vi "main.vi"() -> ()   [LabVIEW 2020]
doc: "This VI is used as the driver for the queue to work. It performs the operations in the queue."
uses:
  Typedef's/Data_Cluster.ctl
  Typedef's/Q_Operations.ctl
  <vilib>/Utility/error.llb/DialogType.ctl
  Typedef's/Bewarage_Out_Level.ctl
  Typedef's/Content_Level.ctl
  <vilib>/Utility/config.llb/NI_LVConfig.lvlib
  Typedef's/Timer_Details.ctl
  Typedef's/Operation_Indication.ctl
  Typedef's/Low_Level_Indications.ctl
  <vilib>/Utility/config.llb/Write Key (I32).vi
  <vilib>/Utility/config.llb/Config Data RefNum.ctl
  <vilib>/Utility/config.llb/Read Key (I32).vi
  <vilib>/Utility/config.llb/Read Key (Boolean).vi
  <vilib>/Utility/config.llb/Read Key (U32).vi
  <vilib>/Utility/config.llb/Write Key (U32).vi
panel:
  out "Error Out":errorcluster
  in  "Error In":errorcluster
  in  "Power":bool
  out "Total Cups":u32
  out "Elapsed Time":i32
  out "Dispensing":bool
  out "Brewing":bool
  out "Grinding":bool
  out "Heating":bool
  out "Purging":bool
  out "Dispenser":i32(slide) min=0 max=60 step=1 scale=0.0..60.0
  out "Chamber":i32(slide) min=0 max=60 step=1 scale=0.0..60.0
  out "Low Milk":bool
  out "Low Bean":bool
  out "Low Water":bool
  out "Milk Level":i32(slide) min=0 max=100 step=1 scale=0.0..100.0
  out "Bean Level":i32(slide) min=0 max=100 step=1 scale=0.0..100.0
  out "Water Level":i32(slide) min=0 max=100 step=1 scale=0.0..100.0
  in  "Bewarage":i32(knob) min=0 max=2 step=1 scale=0.0..2.0
  in  "Carafe":bool
  in  "1 Cup":bool
  # "Description: \n-> Only after power on. Make the button press\nto make coffee"
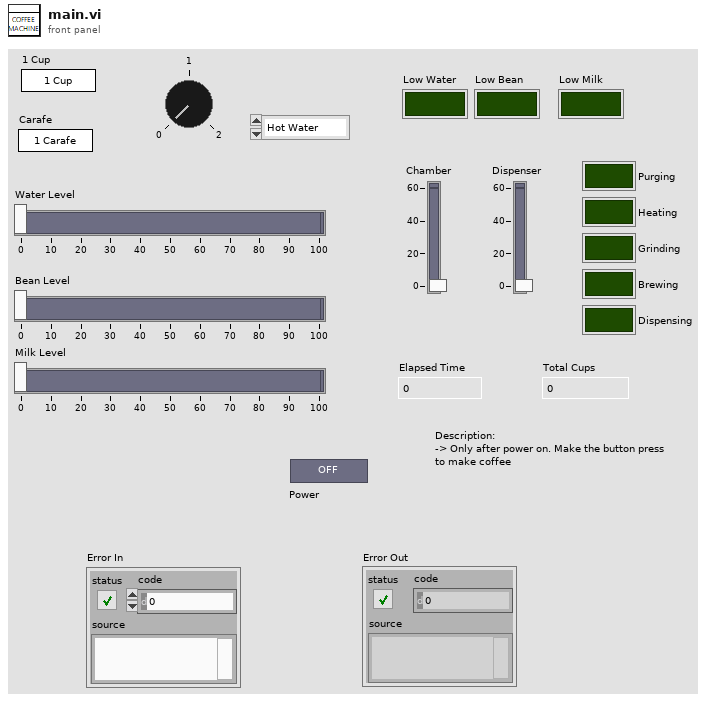
[diagram p1: front panel]
types:
  T1 = typedef "Q_Operations.ctl" = enum16{"Create Q", "Enqueue ", "Dequeue", "Enqueue N ele", "Enstack N ele", "Flush Q", "Destroy Q"}
  T2 = typedef "Data_Cluster.ctl" = cluster{"Cup":bool, "Bewarage":dbl, "Carafe":bool, "Power":bool, "Content Levels":T3, "Beware Out Level":T4, "Timer Operations":T5, "Cups Count":u32, "Bewarage Low Level":i32, "Sequence Array":string[], "Operation Indication":T6, "Bewarage Selection":string, "Low Level Indications":T7, "Config Data Ref":T8}
  T3 = typedef "Content_Level.ctl" = cluster{"Water Level":i32, "Bean Level":i32, "Milk Level":i32}
  T4 = typedef "Bewarage_Out_Level.ctl" = cluster{"Dispenser":i32, "Chamber":i32}
  T5 = typedef "Timer_Details.ctl" = cluster{"Set Time":dbl, "Prev Time":dbl, "Elapsed Time":dbl, "Start?":bool, "Paused?":bool}
  T6 = typedef "Operation_Indication.ctl" = cluster{"Heating":bool, "Grinding":bool, "Dispensing":bool, "Purging":bool, "Brewing":bool}
  T7 = typedef "Low_Level_Indications.ctl" = cluster{"Low Water":bool, "Low Milk":bool, "Low Bean":bool}
  T8 = typedef "NI_LVConfig.lvlib/Config Data RefNum.ctl" = refnum<k1>
  T9 = typedef "DialogType.ctl" = u16
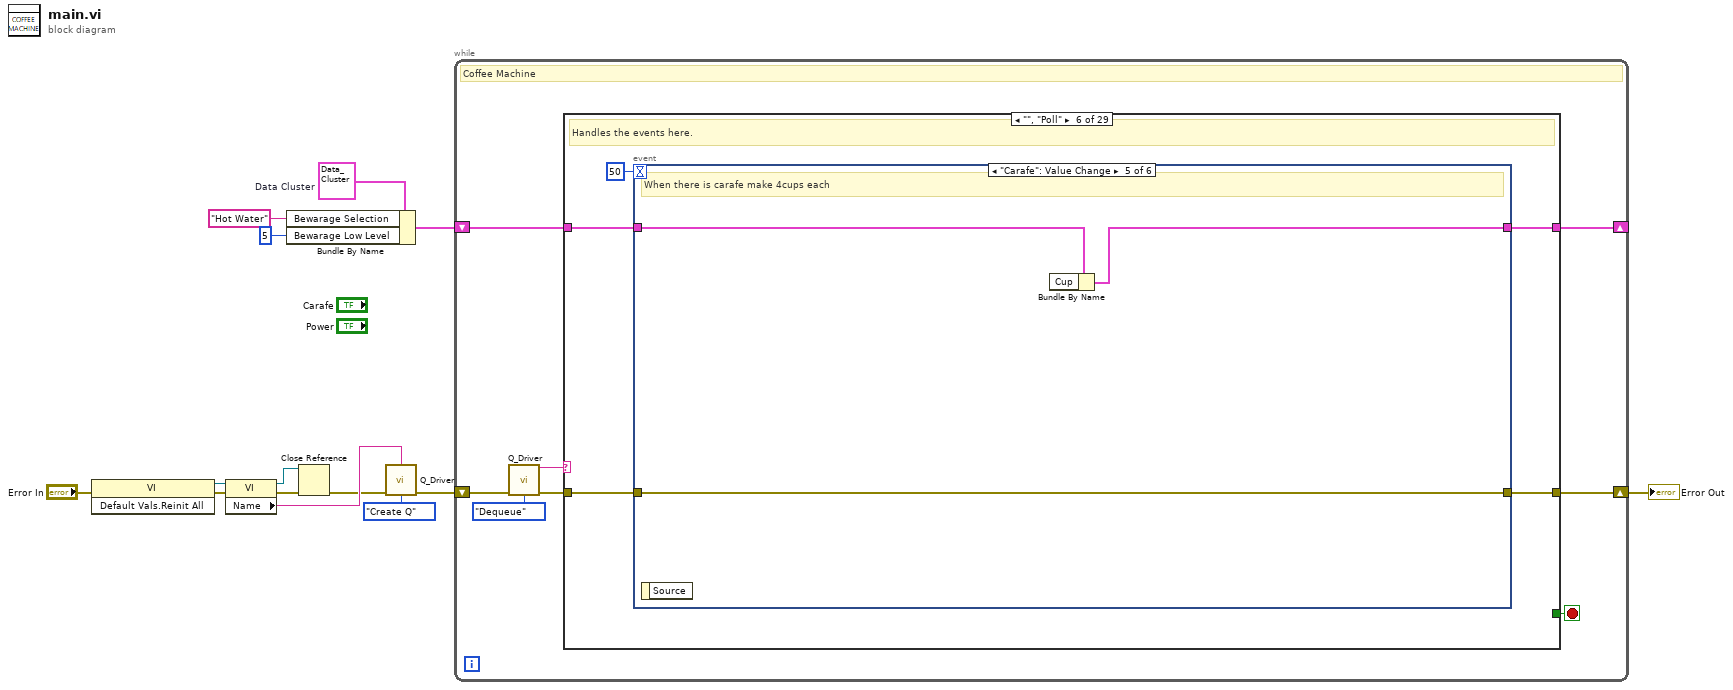
[diagram p0: block diagram]
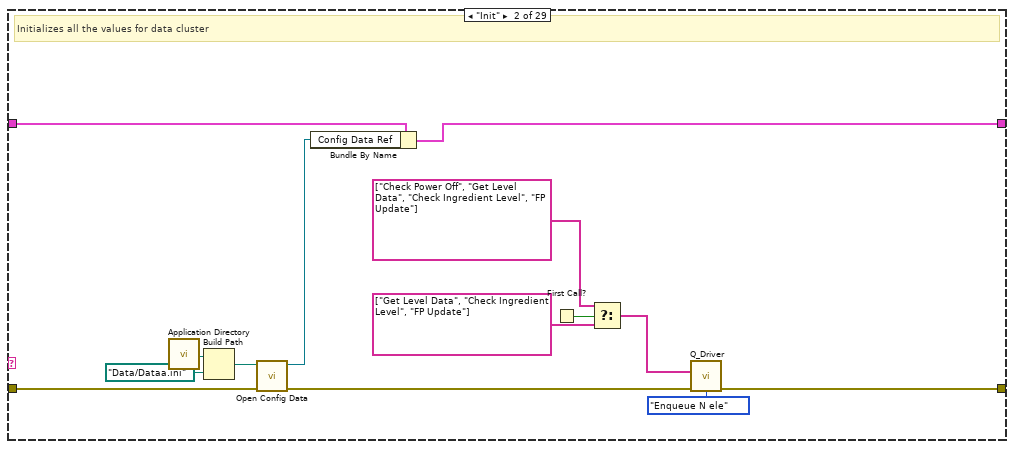
[diagram p3: hidden frame]
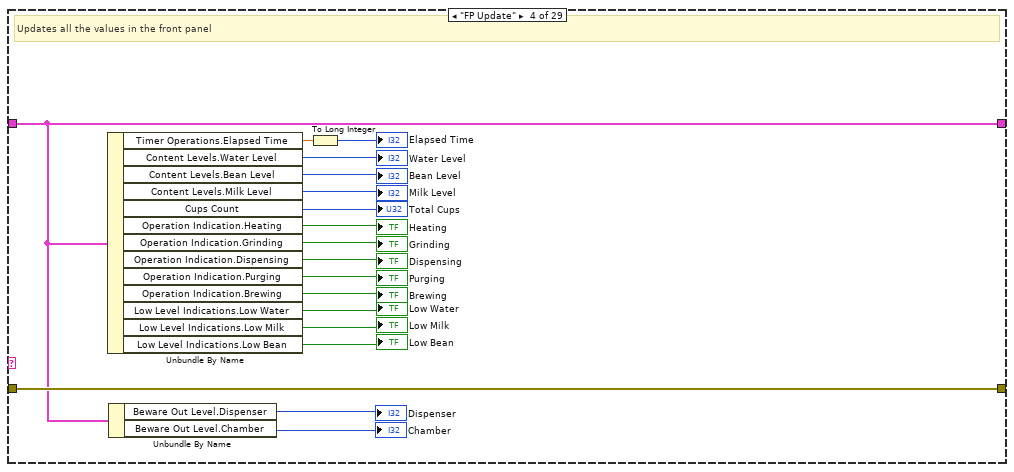
[diagram p5: hidden frame]
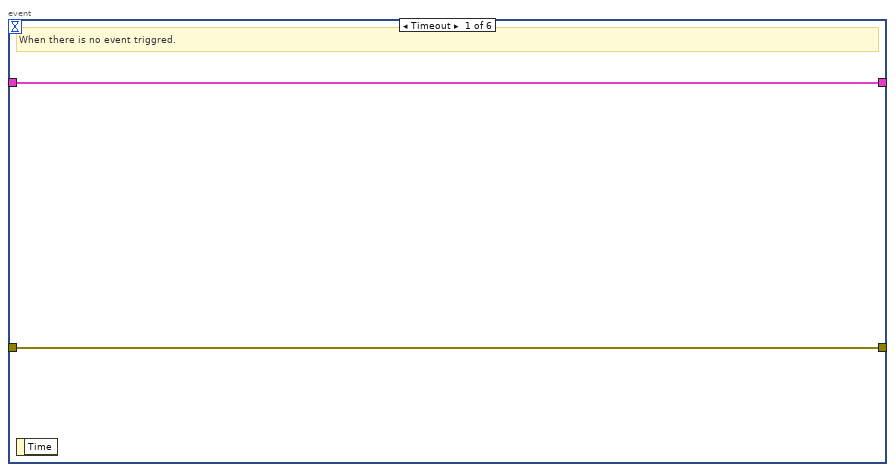
[diagram p7: hidden frame]
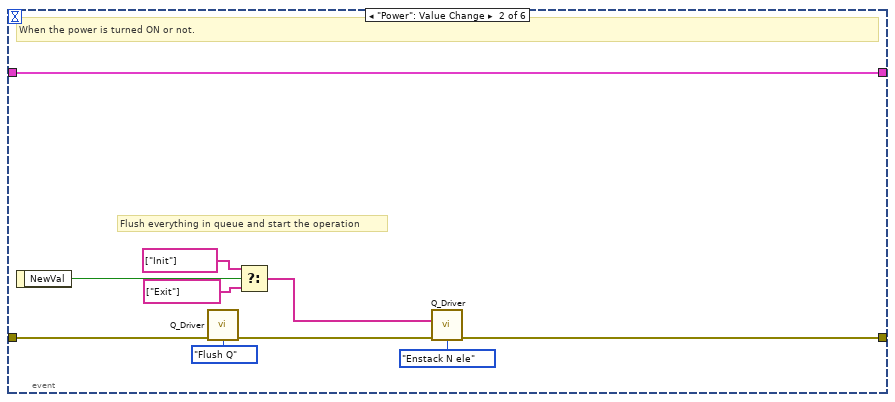
[diagram p8: hidden frame]
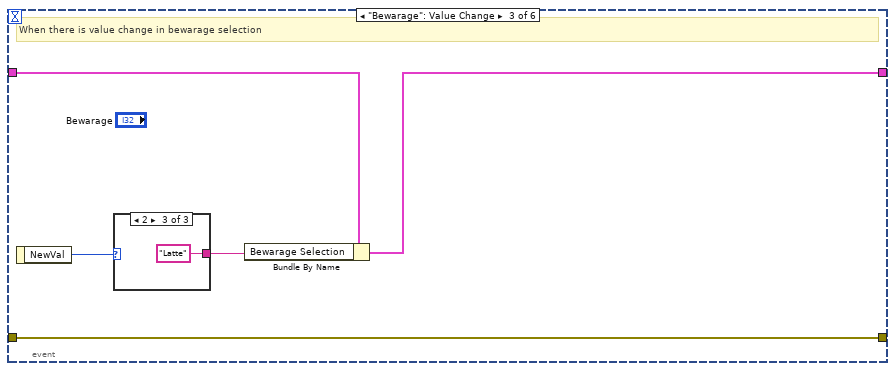
[diagram p9: hidden frame]
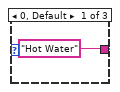
[diagram p10: hidden frame]
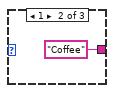
[diagram p11: hidden frame]
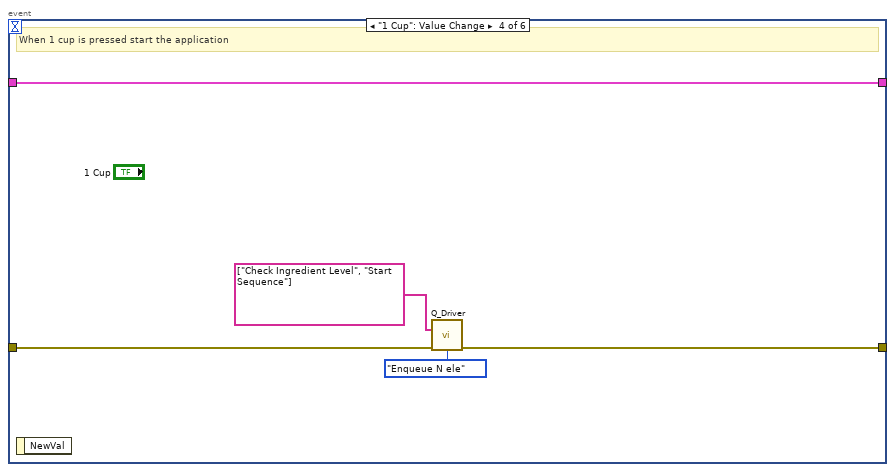
[diagram p12: hidden frame]
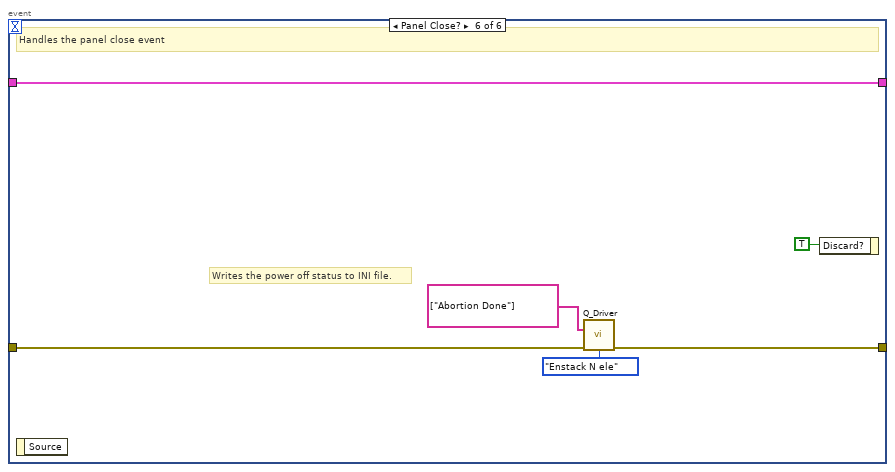
[diagram p13: hidden frame]
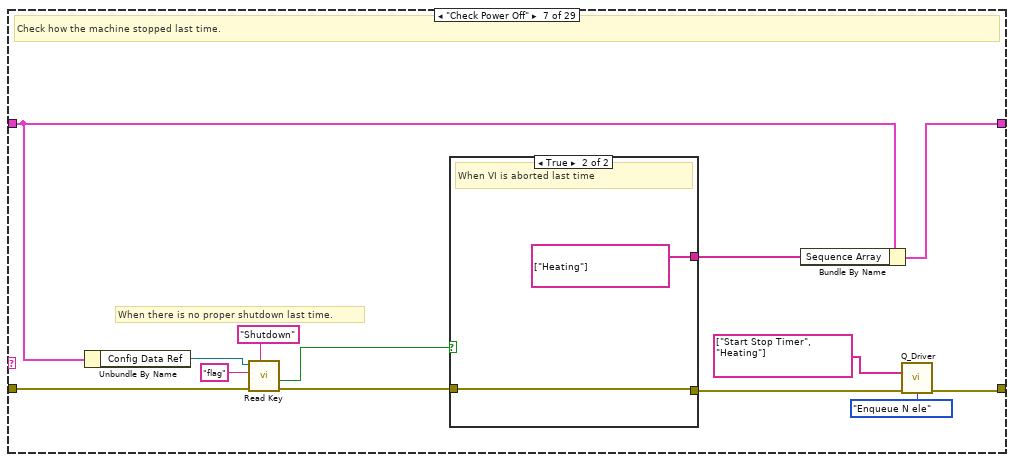
[diagram p14: hidden frame]
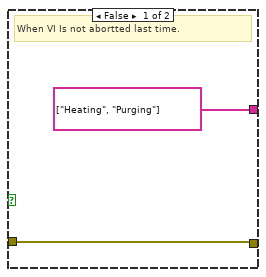
[diagram p15: hidden frame]
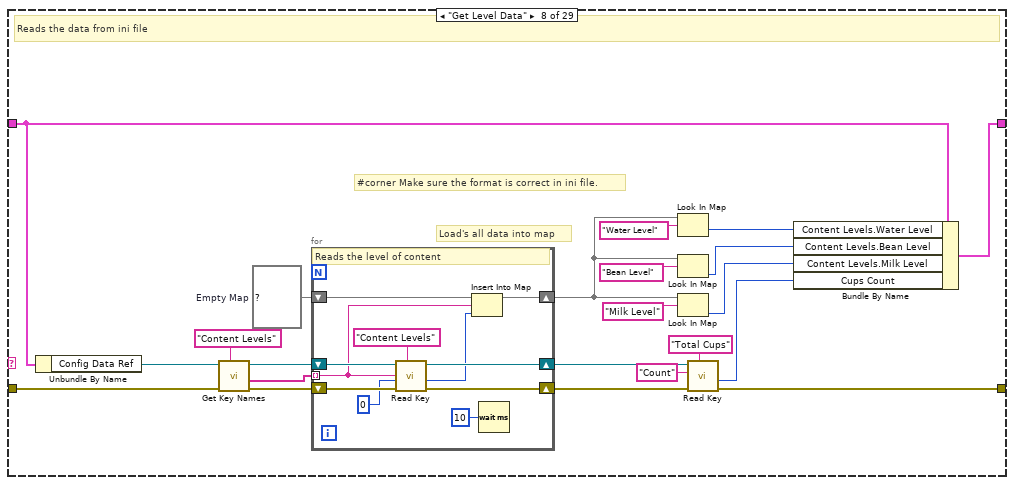
[diagram p16: hidden frame]
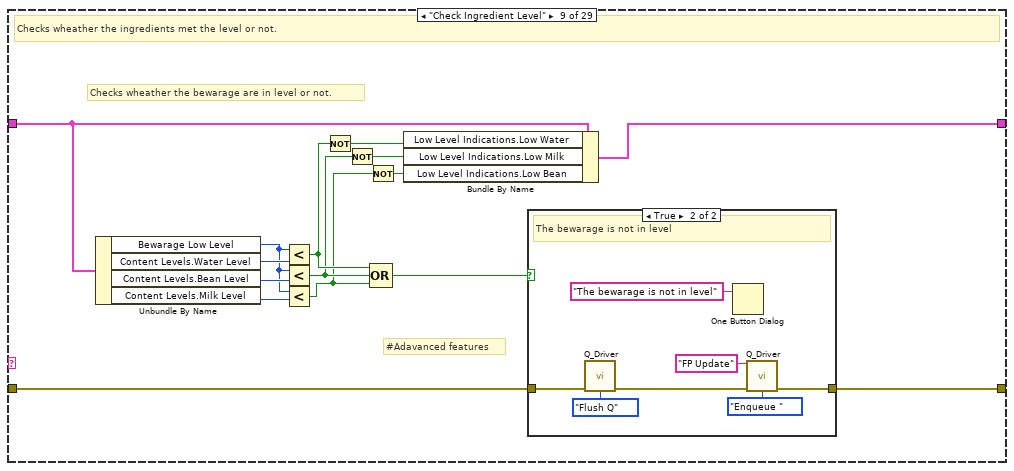
[diagram p17: hidden frame]
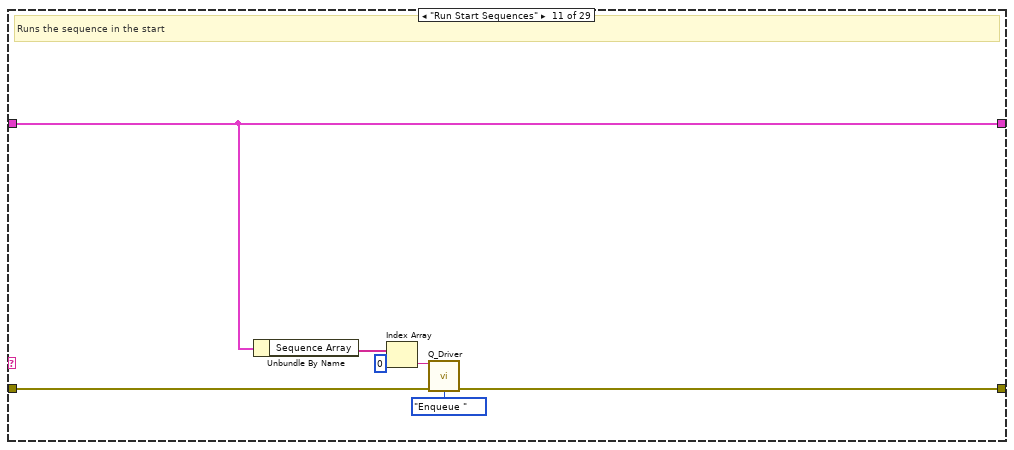
[diagram p20: hidden frame]
diagram:
  w9 = T2 {"Cup"=FALSE, "Bewarage"=0.0, "Carafe"=FALSE, "Power"=FALSE, "Content Levels"={"Water Level"=0, "Bean Level"=0, "Milk Level"=0}, "Beware Out Level"={"Dispenser"=0, "Chamber"=0}, "Timer Operations"={"Set Time"=0.0, "Prev Time"=0.0, "Elapsed Time"=0.0, "Start?"=FALSE, "Paused?"=FALSE}, "Cups Count"=0, "Bewarage Low Level"=30, "Sequence Array"=[], "Operation Indication"={"Heating"=FALSE, "Grinding"=FALSE, "Dispensing"=FALSE, "Purging"=FALSE, "Brewing"=FALSE}, "Bewarage Selection"="Hot Water", "Low Level Indications"={"Low Water"=FALSE, "Low Milk"=FALSE, "Low Bean"=FALSE}, "Config Data Ref"=refnum}  # Data Cluster
  n1 = invoke class="VI" method="Default Vals.Reinit All"(error in="Error In") -> (reference out=w4:refnum<vi>, error out=w5:errorcluster)  [unwired: 2 in, 1 out]
  n2 = property class="VI"(reference=w4, error in=w5) -> (reference out=w2:refnum<vi>, error out=w11:errorcluster, "Name"=w10:string)
  n3 = Bundle By Name(cluster=w9, "Bewarage Selection"="Hot Water", "Bewarage Low Level"=5) -> (w8:T2)
  n4 = Close Reference(reference=w2, error in (no error)=w11) -> (error out=w3:errorcluster)
  n5 = call "Q_Driver.vi"("Q Name"=w10, "Error In"=w3, "Operations"=Q_Operations."Create Q") -> ("Error Out"=w13:errorcluster)  [unwired: 11 in, 1 out]
  n6 = while {
    shift-right: [w21] -> w6
    shift-left: w13 -> [w22]
    shift-right: [w16] -> _
    shift-left: w8 -> [w17]
    stop <- w15 stop-if-true
    # "Coffee Machine"
    n7 = call "Q_Driver.vi"("Error In"=w22, "Operations"=Q_Operations."Dequeue") -> ("Dequeued Ele"=w18:string, "Error Out"=w20:errorcluster)  [unwired: 12 in]
    n8 = case shown="\"\", \"Poll\"" w18 {
      tunnel: w20 -> [w24 w37 w40 w58 w60 w65 w112 w138 w154 w174 w181 w193 w197 w207 w215 w242 w259 w278 w295 w338 w340 w349 w360 w379 w385 w387 w396 w405 w407]
      tunnel: [w24 w36 w40 w58 w60 w64 w102 w122 w153 w174 w177 w191 w198 w207 w210 w237 w258 w277 w290 w310 w340 w349 w351 w379 w382 w387 w390 w400 w407] -> w21
      tunnel: w17 -> [w23 w38 w39 w43 w59 w62 w104 w123 w164 w173 w180 w192 w205 w206 w216 w233 w256 w275 w293 w333 w339 w347 w359 w378 w380 w386 w395 w402 w406]
      tunnel: [w23 w34 w39 w43 w59 w61 w105 w127 w158 w173 w180 w189 w204 w206 w214 w241 w262 w281 w294 w326 w339 w348 w355 w378 w380 w386 w395 w402 w406] -> w16
      tunnel: [_ _ _ _ _ _ _ _ _ _ _ _ _ _ _ _ _ _ _ _ _ _ _ _ _ _ TRUE TRUE _] -> w15
      frame "/**** Initialization ****/" {
      }
      frame "Init" {
        # "Initializes all the values for data cluster"
        n9 = call <vilib>:"Application Directory.vi"() -> ("Application Directory"=w31:path)
        n10 = Build Path(base path=w31, name or relative path=path "Data/Dataa.ini") -> (appended path=w30:path)
        n11 = call <vilib>:"Open Config Data.vi"("error in (no error)"=w37, "configuration file path"=w30) -> ("error out"=w33:errorcluster, "refnum"=w29:T8)  [unwired: 7 in, 1 out]
        n12 = Bundle By Name(cluster=w38, "Config Data Ref"=w29) -> (w34:T2)
        n13 = First Call?() -> (First Call?: T/F=w28:bool)
        n14 = Select(t=string[] ["Check Power Off", "Get Level Data", "Check Ingredient Level", "FP Update"], s=w28, f=string[] ["Get Level Data", "Check Ingredient Level", "FP Update"]) -> (s? t:f=w25:string[])
        n15 = call "Q_Driver.vi"("States[]"=w25, "Error In"=w33, "Operations"=Q_Operations."Enqueue N ele") -> ("Error Out"=w36:errorcluster)  [unwired: 11 in, 1 out]
      }
      frame "/***** FP Related ****/" {
      }
      frame "FP Update" {
        # "Updates all the values in the front panel"
        n16 = Unbundle By Name(w43) -> ("Timer Operations.Elapsed Time"=w48:dbl, "Content Levels.Water Level"=→"Water Level":i32, "Content Levels.Bean Level"=→"Bean Level":i32, "Content Levels.Milk Level"=→"Milk Level":i32, "Cups Count"=→"Total Cups":u32, "Operation Indication.Heating"=→"Heating":bool, "Operation Indication.Grinding"=→"Grinding":bool, "Operation Indication.Dispensing"=→"Dispensing":bool, "Operation Indication.Purging"=→"Purging":bool, "Operation Indication.Brewing"=→"Brewing":bool, "Low Level Indications.Low Water"=→"Low Water":bool, "Low Level Indications.Low Milk"=→"Low Milk":bool, "Low Level Indications.Low Bean"=→"Low Bean":bool)
        n17 = Unbundle By Name(w43) -> ("Beware Out Level.Dispenser"=→"Dispenser":i32, "Beware Out Level.Chamber"=→"Chamber":i32)
        n18 = To Long Integer(number=w48) -> (32bit integer=→"Elapsed Time":i32)
      }
      frame "/***** Events and Functionalities *****/" {
      }
      frame "", "Poll" {
        # "Handles the events here."
        n19 = event shown="[4] \"Carafe\": Value Change" {
          selector: _ -> [_ _ _ _ _ _]
          dyn-events: _ -> [_ _ _ _ _ _]
          timeout: 50 -> [_ _ _ _ _ _]
          tunnel: [w67 w72 w82 w88 w93 w97] -> w64
          tunnel: w65 -> [w67 w77 w82 w90 w93 w99]
          tunnel: [w66 w76 w79 w89 w91 w94] -> w61
          tunnel: w62 -> [w66 w76 w81 w89 w92 w94]
          event Timeout {
            # "When there is no event triggred."
            n20 = event-data() -> ()  [unwired: 1 in, 1 out]
          }
          event "Power": Value Change {
            # "Flush everything in queue and start the operation"
            # "When the power is turned ON or not."
            n21 = event-data() -> ("NewVal"=w75:bool)  [unwired: 1 in]
            n22 = call "Q_Driver.vi"("Error In"=w77, "Operations"=Q_Operations."Flush Q") -> ("Error Out"=w69:errorcluster)  [unwired: 12 in, 1 out]
            n23 = Select(t=string[] ["Init"], s=w75, f=string[] ["Exit"]) -> (s? t:f=w70:string[])
            n24 = call "Q_Driver.vi"("States[]"=w70, "Error In"=w69, "Operations"=Q_Operations."Enstack N ele") -> ("Error Out"=w72:errorcluster)  [unwired: 11 in, 1 out]
          }
          event "Bewarage": Value Change {
            # "When there is value change in bewarage selection"
            n25 = event-data() -> ("NewVal"=w80:i32)  [unwired: 1 in]
            n26 = case shown="2" w80 {
              tunnel: ["Hot Water" "Coffee" "Latte"] -> w78
              frame 0, Default {
              }
              frame 1 {
              }
              frame 2 {
              }
            }
            n27 = Bundle By Name(cluster=w81, "Bewarage Selection"=w78) -> (w79:T2)
          }
          event "1 Cup": Value Change {
            # "When 1 cup is pressed start the application"
            n28 = event-data() -> ()  [unwired: 1 in, 1 out]
            n29 = call "Q_Driver.vi"("States[]"=string[] ["Check Ingredient Level", "Start Sequence"], "Error In"=w90, "Operations"=Q_Operations."Enqueue N ele") -> ("Error Out"=w88:errorcluster)  [unwired: 11 in, 1 out]
          }
          event "Carafe": Value Change {
            # "When there is carafe make 4cups each"
            n30 = event-data() -> ()  [unwired: 1 in, 1 out]
            n31 = Bundle By Name(cluster=w92) -> (w91:T2)  [unwired: 1 in]
          }
          event Panel Close? {
            # "Writes the power off status to INI file."
            # "Handles the panel close event"
            n32 = event-data() -> ()  [unwired: 1 in, 1 out]
            n33 = call "Q_Driver.vi"("States[]"=string[] ["Abortion Done"], "Error In"=w99, "Operations"=Q_Operations."Enstack N ele") -> ("Error Out"=w97:errorcluster)  [unwired: 11 in, 1 out]
            n34 = event-data("Discard?"=TRUE) -> ()  [unwired: 1 in, 1 out]
          }
        }
      }
      frame "Check Power Off" {
        # "When there is no proper shutdown last time."
        # "Check how the machine stopped last time."
        n35 = Unbundle By Name(w104) -> ("Config Data Ref"=w108:T8)
        n36 = call-poly <vilib>:"Read Key.vi"("section"="Shutdown", "error in (no error)"=w112, "key"="flag", "refnum"=w108) -> ("error out"=w107:errorcluster, "value"=w109:bool)  [unwired: 4 in, 2 out]
        n37 = case shown="True" w109 {
          tunnel: [w114 w116] -> w106
          tunnel: w107 -> [w114 w116]
          tunnel: [string[] ["Heating", "Purging"] ("Sequence Array") string[] ["Heating"] ("Sequence Array")] -> w103
          frame False {
            # "When VI Is not abortted last time."
          }
          frame True {
            # "When VI is aborted last time"
          }
        }
        n38 = Bundle By Name(cluster=w104, "Sequence Array"=w103) -> (w105:T2)
        n39 = call "Q_Driver.vi"("States[]"=string[] ["Start Stop Timer", "Heating"], "Error In"=w106, "Operations"=Q_Operations."Enqueue N ele") -> ("Error Out"=w102:errorcluster)  [unwired: 11 in, 1 out]
      }
      frame "Get Level Data" {
        w133 = map{string, i32} {}  # Empty Map
        # "Load's all data into map"
        # "#corner Make sure the format is correct in ini file."
        # "Reads the data from ini file"
        n40 = Unbundle By Name(w123) -> ("Config Data Ref"=w117:T8)
        n41 = call <vilib>:"Get Key Names.vi"("section"="Content Levels", "error in (no error)"=w138, "refnum"=w117) -> ("error out"=w137:errorcluster, "key names"=w135:string[], "refnum out"=w134:T8)  [unwired: 5 in, 1 out]
        n42 = for {
          shift-right: [w148] -> w136
          shift-left: w137 -> [w149]
          tunnel: w135 -> [w142] mode=indexing
          shift-right: [w145] -> w121
          shift-left: w134 -> [w146]
          shift-right: [w140] -> w128
          shift-left: w133 -> [w143]
          # "Reads the level of content"
          n43 = call-poly <vilib>:"Read Key.vi"("section"="Content Levels", "error in (no error)"=w149, "default value"=0, "key"=w142, "refnum"=w146) -> ("error out"=w148:errorcluster, "value"=w141:i32, "refnum out"=w145:T8)  [unwired: 3 in, 1 out]
          n44 = Insert Into Map(map in=w143, key=w142, value=w141) -> (map out=w140:map{string, i32})  [unwired: 2 out]
          n45 = Wait (ms)(milliseconds to wait=u32 10) -> ()  [unwired: 1 out]
        }
        n46 = Look In Map(map=w128, key="Water Level") -> (value=w126:i32)  [unwired: 1 in, 1 out]
        n47 = Look In Map(map=w128, key="Bean Level") -> (value=w125:i32)  [unwired: 1 in, 1 out]
        n48 = Look In Map(map=w128, key="Milk Level") -> (value=w124:i32)  [unwired: 1 in, 1 out]
        n49 = call-poly <vilib>:"Read Key.vi"("section"="Total Cups", "error in (no error)"=w136, "key"="Count", "refnum"=w121) -> ("error out"=w122:errorcluster, "value"=w120:u32)  [unwired: 4 in, 2 out]
        n50 = Bundle By Name(cluster=w123, "Content Levels.Water Level"=w126, "Content Levels.Bean Level"=w125, "Content Levels.Milk Level"=w124, "Cups Count"=w120) -> (w127:T2)
      }
      frame "Check Ingredient Level" {
        # "#Adavanced features"
        # "Checks wheather the bewarage are in level or not."
        # "Checks wheather the ingredients met the level or not."
        n51 = Unbundle By Name(w164) -> ("Bewarage Low Level"=w160:i32, "Content Levels.Water Level"=w163:i32, "Content Levels.Bean Level"=w162:i32, "Content Levels.Milk Level"=w161:i32)
        n52 = Less?(x=w160, y=w163) -> (x < y?=w157:bool)
        n53 = Less?(x=w160, y=w162) -> (x < y?=w156:bool)
        n54 = Less?(x=w160, y=w161) -> (x < y?=w155:bool)
        n55 = Not(x=w157) -> (.not. x?=w152:bool)
        n56 = Not(x=w156) -> (.not. x?=w151:bool)
        n57 = Not(x=w155) -> (.not. x?=w150:bool)
        n58 = Compound Arithmetic op=OR(w157, w156, w155) -> (w159:bool)
        n59 = Bundle By Name(cluster=w164, "Low Level Indications.Low Water"=w152, "Low Level Indications.Low Milk"=w151, "Low Level Indications.Low Bean"=w150) -> (w158:T2)
        n60 = case shown="True" w159 {
          tunnel: w154 -> [w165 w171]
          tunnel: [w165 w168] -> w153
          frame False {
            # "When they are in level"
          }
          frame True {
            # "The bewarage is not in level"
            n61 = call "Q_Driver.vi"("Error In"=w171, "Operations"=Q_Operations."Flush Q") -> ("Error Out"=w170:errorcluster)  [unwired: 12 in, 1 out]
            n62 = One Button Dialog(message="The bewarage is not in level") -> ()  [unwired: 1 in, 1 out]
            n63 = call "Q_Driver.vi"("State"="FP Update", "Error In"=w170, "Operations"=Q_Operations."Enqueue ") -> ("Error Out"=w168:errorcluster)  [unwired: 11 in, 1 out]
          }
        }
      }
      frame "/***** Start Sequence Runners ****/" {
      }
      frame "Run Start Sequences" {
        # "Runs the sequence in the start"
        n64 = Unbundle By Name(w180) -> ("Sequence Array"=w179:string[])
        n65 = Index Array(array=w179, index=0) -> (element=w176:string)
        n66 = call "Q_Driver.vi"("State"=w176, "Error In"=w181, "Operations"=Q_Operations."Enqueue ") -> ("Error Out"=w177:errorcluster)  [unwired: 11 in, 1 out]
      }
      frame "Heating" {
        # "Heating Process"
        n67 = Bundle By Name(cluster=T6 {"Heating"=FALSE, "Grinding"=FALSE, "Dispensing"=FALSE, "Purging"=FALSE, "Brewing"=FALSE} ("Operation Indication"), "Heating"=TRUE) -> (w188:T6)
        n68 = Get Date/Time In Seconds() -> (seconds since 1Jan1904=w183:timestamp)
        n69 = To Double Precision Float(number=w183) -> (double precision float=w182:dbl)
        n70 = Bundle By Name(cluster=w192, "Operation Indication"=w188, "Timer Operations.Set Time"=5.0, "Timer Operations.Prev Time"=w182) -> (w189:T2)
        n71 = call "Q_Driver.vi"("State"="Get Elapsed Time", "Error In"=w193, "Operations"=Q_Operations."Enqueue ") -> ("Error Out"=w191:errorcluster)  [unwired: 11 in, 1 out]
      }
      frame "Purging" {
        # "Purging process to be done"
        n72 = Get Date/Time In Seconds() -> (seconds since 1Jan1904=w195:timestamp)
        n73 = Bundle By Name(cluster=T6 {"Heating"=FALSE, "Grinding"=FALSE, "Dispensing"=FALSE, "Purging"=FALSE, "Brewing"=FALSE} ("Operation Indication"), "Purging"=TRUE) -> (w201:T6)
        n74 = To Double Precision Float(number=w195) -> (double precision float=w194:dbl)
        n75 = Bundle By Name(cluster=w205, "Operation Indication"=w201, "Timer Operations.Set Time"=4.0, "Timer Operations.Prev Time"=w194) -> (w204:T2)
        n76 = call "Q_Driver.vi"("State"="Get Elapsed Time", "Error In"=w197, "Operations"=Q_Operations."Enqueue ") -> ("Error Out"=w198:errorcluster)  [unwired: 11 in, 1 out]
      }
      frame "/**** Sequence Runners ****/" {
        # "States to run the sequences."
      }
      frame "Start Sequence" {
        # "Starts the sequence by updating things into tthe array"
        n77 = Unbundle By Name(w216) -> ("Bewarage Selection"=w217:string)
        n78 = case shown="\"Latte\"" w217 {
          tunnel: w216 -> [_ _ _ _]
          tunnel: w215 -> [w219 w220 w223 w225]
          tunnel: [w219 w220 w223 w225] -> w209
          tunnel: [string[] ["Dispensing"] string[] ["Grinding", "Brewing", "Dispensing"] string[] ["Grinding", "Brewing", "Dispensing"] string[] []] -> w208
          frame "Hot Water" {
          }
          frame "Coffee" {
          }
          frame "Latte" {
          }
          frame Default {
          }
        }
        n79 = Index Array(array=w208, index=0) -> (element=w213:string)
        n80 = call "Q_Driver.vi"("State"=w213, "Error In"=w209, "Operations"=Q_Operations."Enqueue ") -> ("Error Out"=w210:errorcluster)  [unwired: 11 in, 1 out]
        n81 = Bundle By Name(cluster=w216, "Sequence Array"=w208) -> (w214:T2)
      }
      frame "Grinding" {
        w230 = 5 ("y")
        # "Runs the grinding sequence."
        n82 = Unbundle By Name(w233) -> ("Content Levels.Bean Level"=w232:i32, "Beware Out Level.Chamber"=w228:i32)
        n83 = Subtract(x=w232, y=w230) -> (x-y=w231:i32)
        n84 = Add(x=w230, y=w228) -> (x+y=w229:i32)
        n85 = call "Q_Driver.vi"("State"="Get Elapsed Time", "Error In"=w242, "Operations"=Q_Operations."Enqueue ") -> ("Error Out"=w237:errorcluster)  [unwired: 11 in, 1 out]
        n86 = Bundle By Name(cluster=T6 {"Heating"=FALSE, "Grinding"=FALSE, "Dispensing"=FALSE, "Purging"=FALSE, "Brewing"=FALSE} ("Operation Indication"), "Grinding"=TRUE) -> (w239:T6)
        n87 = Get Date/Time In Seconds() -> (seconds since 1Jan1904=w227:timestamp)
        n88 = To Double Precision Float(number=w227) -> (double precision float=w226:dbl)
        n89 = Bundle By Name(cluster=w233, "Operation Indication"=w239, "Timer Operations.Set Time"=3.0, "Content Levels.Bean Level"=w231, "Beware Out Level.Chamber"=w229, "Timer Operations.Prev Time"=w226) -> (w241:T2)
      }
      frame "Brewing" {
        n90 = Unbundle By Name(w256) -> ("Content Levels.Milk Level"=w255:i32, "Beware Out Level.Chamber"=w245:i32, "Bewarage Selection"=w251:string)
        n91 = Equal?(x=w251, y="Coffee") -> (x = y?=w249:bool)
        n92 = Select(t=0, s=w249, f=5) -> (s? t:f=w246:i32)
        n93 = Add(x=w245, y=w246) -> (x+y=w252:i32)
        n94 = Subtract(x=w255, y=5) -> (x-y=w254:i32)
        n95 = call "Q_Driver.vi"("State"="Get Elapsed Time", "Error In"=w259, "Operations"=Q_Operations."Enqueue ") -> ("Error Out"=w258:errorcluster)  [unwired: 11 in, 1 out]
        n96 = Bundle By Name(cluster=T6 {"Heating"=FALSE, "Grinding"=FALSE, "Dispensing"=FALSE, "Purging"=FALSE, "Brewing"=FALSE} ("Operation Indication"), "Brewing"=TRUE ("Grinding")) -> (w264:T6)
        n97 = Get Date/Time In Seconds() -> (seconds since 1Jan1904=w244:timestamp)
        n98 = To Double Precision Float(number=w244) -> (double precision float=w243:dbl)
        n99 = Bundle By Name(cluster=w256, "Operation Indication"=w264, "Timer Operations.Set Time"=4.0, "Content Levels.Milk Level"=w254, "Beware Out Level.Chamber"=w252, "Timer Operations.Prev Time"=w243) -> (w262:T2)
      }
      frame "Dispensing" {
        w272 = 5 ("y")
        n100 = Unbundle By Name(w275) -> ("Content Levels.Water Level"=w274:i32, "Beware Out Level.Dispenser"=w271:i32, "Beware Out Level.Chamber"=w269:i32)
        n101 = Subtract(x=w274, y=w272) -> (x-y=w273:i32)
        n102 = Bundle By Name(cluster=T6 {"Heating"=FALSE, "Grinding"=FALSE, "Dispensing"=FALSE, "Purging"=FALSE, "Brewing"=FALSE} ("Operation Indication"), "Dispensing"=TRUE ("Grinding")) -> (w283:T6)
        n103 = Get Date/Time In Seconds() -> (seconds since 1Jan1904=w267:timestamp)
        n104 = Compound Arithmetic op=ADD(w272, w271, w269) -> (w270:i32)
        n105 = call "Q_Driver.vi"("State"="Get Elapsed Time", "Error In"=w278, "Operations"=Q_Operations."Enqueue ") -> ("Error Out"=w277:errorcluster)  [unwired: 11 in, 1 out]
        n106 = To Double Precision Float(number=w267) -> (double precision float=w266:dbl)
        n107 = Bundle By Name(cluster=w275, "Operation Indication"=w283, "Timer Operations.Set Time"=5.0, "Content Levels.Water Level"=w273, "Beware Out Level.Dispenser"=w270, "Beware Out Level.Chamber"=0, "Timer Operations.Prev Time"=w266) -> (w281:T2)
      }
      frame "Go To Next Sequence" {
        # "Once one sequence is finished run's the next sequence."
        n108 = Unbundle By Name(w293) -> ("Sequence Array"=w292:string[])
        n109 = Delete From Array(array=w292, index=0) -> (array with subset deleted=w287:string[])  [unwired: 1 in, 1 out]
        n110 = Index Array(array=w287, index=0) -> (element=w285:string)
        n111 = Empty Array?(array=w287) -> (empty?=w289:bool)
        n112 = case shown="False" w289 {
          tunnel: w295 -> [w299 w303]
          tunnel: [w298 w302] -> w290
          tunnel: w285 -> [w297 _]
          frame False {
            # "Operate next seq"
            n113 = call "Q_Driver.vi"("State"=w297, "Error In"=w299, "Operations"=Q_Operations."Enqueue ") -> ("Error Out"=w298:errorcluster)  [unwired: 11 in, 1 out]
          }
          frame True {
            # "Operation finished"
            n114 = call "Q_Driver.vi"("State"="Operation Finished", "Error In"=w303, "Operations"=Q_Operations."Enqueue ") -> ("Error Out"=w302:errorcluster)  [unwired: 11 in, 1 out]
          }
        }
        n115 = Bundle By Name(cluster=w293, "Sequence Array"=w287, "Timer Operations.Elapsed Time"=0.0) -> (w294:T2)
      }
      frame "Operation Finished" {
        w307 = 0 ("Beware Out Level.Dispenser")
        w315 = "Content Levels" ("section")
        # "Finished running operation"
        n116 = Unbundle By Name(w333) -> ("Cups Count"=w332:u32, "Config Data Ref"=w331:T8)
        n117 = call "Q_Driver.vi"("States[]"=string[] ["FP Update"], "Error In"=w338, "Operations"=Q_Operations."Enqueue N ele") -> ("Error Out"=w336:errorcluster)  [unwired: 11 in, 1 out]
        n118 = Increment(x=w332) -> (x+1=w327:u32)
        n119 = Bundle By Name(cluster=w333, "Operation Indication"=T6 {"Heating"=FALSE, "Grinding"=FALSE, "Dispensing"=FALSE, "Purging"=FALSE, "Brewing"=FALSE}, "Cups Count"=w327, "Beware Out Level.Dispenser"=w307, "Beware Out Level.Chamber"=w307) -> (w326:T2)
        n120 = Unbundle By Name(w326) -> ("Content Levels.Water Level"=w324:i32, "Content Levels.Bean Level"=w320:i32, "Content Levels.Milk Level"=w313:i32)
        n121 = call-poly <vilib>:"Write Key.vi"("section"="Total Cups", "error in (no error)"=w336, "value"=w327, "key"="count", "refnum"=w331) -> ("error out"=w330:errorcluster, "refnum out"=w318:T8)  [unwired: 4 in, 1 out]
        n122 = call-poly <vilib>:"Write Key.vi"("section"=w315, "error in (no error)"=w330, "value"=w324, "key"="Water Level", "refnum"=w318) -> ("error out"=w322:errorcluster, "refnum out"=w317:T8)  [unwired: 4 in, 1 out]
        n123 = call-poly <vilib>:"Write Key.vi"("section"=w315, "error in (no error)"=w322, "value"=w320, "key"="Bean Level", "refnum"=w317) -> ("error out"=w321:errorcluster, "refnum out"=w316:T8)  [unwired: 4 in, 1 out]
        n124 = call-poly <vilib>:"Write Key.vi"("section"=w315, "error in (no error)"=w321, "value"=w313, "key"="Milk Level", "refnum"=w316) -> ("error out"=w319:errorcluster, "refnum out"=w305:T8)  [unwired: 4 in, 1 out]
        n125 = call <vilib>:"Close Config Data.vi"("error in (no error)"=w319, "write file if changed (T)"=TRUE, "refnum"=w305) -> ("error out"=w306:errorcluster)  [unwired: 7 in, 1 out]
        n126 = call "Q_Driver.vi"("Error In"=w306, "Operations"=Q_Operations."Flush Q") -> ("Error Out"=w312:errorcluster)  [unwired: 12 in, 1 out]
        n127 = call "Q_Driver.vi"("State"="Init", "Error In"=w312, "Operations"=Q_Operations."Enqueue ") -> ("Error Out"=w310:errorcluster)  [unwired: 11 in, 1 out]
      }
      frame "/**** Timer Operations ****/" {
      }
      frame "Start Stop Timer" {
        # "Starts the timer"
        n128 = Unbundle By Name(w347) -> ("Timer Operations.Start?"=w346:bool)
        n129 = Get Date/Time In Seconds() -> (seconds since 1Jan1904=w344:timestamp)
        n130 = To Double Precision Float(number=w344) -> (double precision float=w342:dbl)
        n131 = Not(x=w346) -> (.not. x?=w345:bool)
        n132 = Bundle By Name(cluster=w347, "Timer Operations.Start?"=w345, "Timer Operations.Set Time"=0.0, "Timer Operations.Prev Time"=w342, "Timer Operations.Paused?"=FALSE) -> (w348:T2)
      }
      frame "Get Elapsed Time" {
        # "When set point is reached"
        # "Get's the elapsed time between the runs."
        n133 = Unbundle By Name(w359) -> ("Timer Operations.Paused?"=w358:bool, "Timer Operations.Prev Time"=w357:dbl, "Timer Operations.Elapsed Time"=w356:dbl, "Timer Operations.Set Time"=w353:dbl)
        n134 = case shown="False" w358 {
          tunnel: w357 -> [w372 _]
          tunnel: w356 -> [w370 w375]
          tunnel: [w373 w376] -> w354
          tunnel: [w371 w375] -> w352
          frame False {
            # "When timer is paused"
            n135 = Get Date/Time In Seconds() -> (seconds since 1Jan1904=w374:timestamp)
            n136 = To Double Precision Float(number=w374) -> (double precision float=w373:dbl)
            n137 = Subtract(x=w373, y=w372) -> (x-y=w369:dbl)
            n138 = Add(x=w369, y=w370) -> (x+y=w371:dbl)
          }
          frame True {
            # "When timer is not paused"
            n139 = Get Date/Time In Seconds() -> (seconds since 1Jan1904=w377:timestamp)
            n140 = To Double Precision Float(number=w377) -> (double precision float=w376:dbl)
          }
        }
        n141 = Greater?(x=w352, y=w353) -> (0:w350:bool)
        n142 = case shown="False" w350 {
          tunnel: w360 -> [w364 w368]
          tunnel: [w363 w367] -> w351
          frame False {
            # "Doesn't reached setpoint"
            n143 = call "Q_Driver.vi"("States[]"=string[] ["Get Elapsed Time", "FP Update", "Poll"] ("State"), "Error In"=w364, "Operations"=Q_Operations."Enqueue N ele") -> ("Error Out"=w363:errorcluster)  [unwired: 11 in, 1 out]
          }
          frame True {
            # "REached set point"
            n144 = call "Q_Driver.vi"("States[]"=string[] ["Go To Next Sequence"], "Error In"=w368, "Operations"=Q_Operations."Enqueue N ele") -> ("Error Out"=w367:errorcluster)  [unwired: 11 in, 1 out]
          }
        }
        n145 = Bundle By Name(cluster=w359, "Timer Operations.Prev Time"=w354, "Timer Operations.Elapsed Time"=w352) -> (w355:T2)
      }
      frame "/**** Errors *****/" {
      }
      frame "Error" {
        w383 = T9 2 items=["no dialog", "OK message", "continue or stop message", "OK message + warnings", "continue/stop + warnings"] ("type of dialog (OK msg:1)")
        # "Just pop up the errror"
        # "Handle the error's here"
        n146 = call <vilib>:"Simple Error Handler.vi"("type of dialog (OK msg:1)"=w383, "error in (no error)"=w385) -> ("code out"=w381:i32, "error out"=w384:errorcluster)  [unwired: 3 in, 3 out]
        n147 = call <vilib>:"Clear Errors.vi"("error in (no error)"=w384, "specific error code to clear (0: all)"=w381) -> ("error out"=w382:errorcluster)  [unwired: 4 in, 1 out]
      }
      frame "/ ***** Exit ***** /" {
      }
      frame "Abortion Done" {
        # "Aborting the VI has done. Write the data into ini file"
        n148 = Unbundle By Name(w395) -> ("Config Data Ref"=w391:T8)
        n149 = call "Write_Power_Off_Status.vi"("Config File Ref"=w391, "Value"=TRUE, "error in (no error)"=w396) -> ("Config File Ref Out"=w389:T8, "error out"=w394:errorcluster)  [unwired: 11 in]
        n150 = call <vilib>:"Close Config Data.vi"("error in (no error)"=w394, "write file if changed (T)"=FALSE, "refnum"=w389) -> ("error out"=w390:errorcluster)  [unwired: 7 in, 1 out]
      }
      frame "Exit" {
        # "Writes the status of power off in the ini file."
        # "Handles operations during exit"
        n151 = Unbundle By Name(w402) -> ("Config Data Ref"=w398:T8)
        n152 = call "Write_Power_Off_Status.vi"("Config File Ref"=w398, "Value"=FALSE, "error in (no error)"=w405) -> ("Config File Ref Out"=w397:T8, "error out"=w403:errorcluster)  [unwired: 11 in]
        n153 = call <vilib>:"Close Config Data.vi"("error in (no error)"=w403, "write file if changed (T)"=TRUE, "refnum"=w397) -> ("error out"=w400:errorcluster)  [unwired: 7 in, 1 out]
      }
      frame "Developer Error", Default {
        # "Mistakes done by developer"
      }
    }
  }
  "Error Out" <- w6
